vi "Main_20A.vi"() -> ()   [LabVIEW 2024]
uses:
  Utility/Universal Utility/TypeDefs_Utility/Cluster_Row-Column.ctl
  9e3f57c0-2ef8-4495-8287-c6a42a5fb955.vi
  Utility/Universal Utility/TypeDefs_Utility/ENUM_4 Directions U-D-L-R.ctl
  Utility/Universal Utility/TypeDefs_Utility/ENUM_8 Directions U-D-L-R.ctl
panel:
  in  "Select Data":enum32{"Example", "Puzzle"}(tab)
  in  "Example":string="###############\n#...#...#.....#\n#.#.#.#.#.###.#\n#S#...#.#.#...#\n#######.#.#.###\n#######.#.#...#\n#######.#.###.#\n###..E#...#...#\n###.#######.###\n#...###...#...#\n#.#####.#.###.#\n#.#...#.#.#...#\n#.#.#.#.#.#.###\n#...#...#...###\n###############"
  in  "Puzzle":string="#############################################################################################################################################\n#...............#...#...#.......#...#.........###...#...#.....#...#...........#...###.....###.....#.....#...###.........#...#...#...###.....#\n#.#############.#.#.#.#.#.#####.#.#.#.#######.###.#.#.#.#.###.#.#.#.#########.#.#.###.###.###.###.#.###.#.#.###.#######.#.#.#.#.#.#.###.###.#\n#.....#.......#.#.#...#.#.....#...#.#...#.....#...#.#.#...#...#.#.#.......#...#.#...#...#.#...#...#.#...#.#.#...#.......#.#.#.#.#.#...#...#.#\n#####.#.#####.#.#.#####.#####.#####.###.#.#####.###.#.#####.###.#.#######.#.###.###.###.#.#.###.###.#.###.#.#.###.#######.#.#.#.#.###.###.#.#\n#...#...#.....#...#...#.#...#.....#...#.#.....#...#...#.....#...#...###...#...#...#...#.#.#...#...#.#.#...#.#...#.....###.#.#.#...#...#...#.#\n#.#.#####.#########.#.#.#.#.#####.###.#.#####.###.#####.#####.#####.###.#####.###.###.#.#.###.###.#.#.#.###.###.#####.###.#.#.#####.###.###.#\n#.#.#...#.....#...#.#.#...#.#...#.#...#.....#...#...#...#...#.....#...#.....#...#.#...#.#.###...#.#.#...#...#...#.....#...#.#.#.....###...#.#\n#.#.#.#.#####.#.#.#.#.#####.#.#.#.#.#######.###.###.#.###.#.#####.###.#####.###.#.#.###.#.#####.#.#.#####.###.###.#####.###.#.#.#########.#.#\n#.#...#.#...#...#...#.....#.#.#.#.#.#...#...#...#...#...#.#.#.....#...###...#...#.#...#.#.#...#.#...#...#.#...#...#...#...#.#.#...#...#...#.#\n#.#####.#.#.#############.#.#.#.#.#.#.#.#.###.###.#####.#.#.#.#####.#####.###.###.###.#.#.#.#.#.#####.#.#.#.###.###.#.###.#.#.###.#.#.#.###.#\n#...#...#.#.#...#.....#...#...#...#.#.#.#...#...#.#...#...#.#...#...#...#.#...#...#...#.#.#.#.#.....#.#...#...#.###.#...#.#.#.#...#.#...#...#\n###.#.###.#.#.#.#.###.#.###########.#.#.###.###.#.#.#.#####.###.#.###.#.#.#.###.###.###.#.#.#.#####.#.#######.#.###.###.#.#.#.#.###.#####.###\n#...#.#...#.#.#.#...#.#...........#.#.#.###.#...#.#.#.......#...#...#.#.#.#.#...#...###.#.#.#.#...#.#...#.....#...#...#.#.#...#...#.....#...#\n#.###.#.###.#.#.###.#.###########.#.#.#.###.#.###.#.#########.#####.#.#.#.#.#.###.#####.#.#.#.#.#.#.###.#.#######.###.#.#.#######.#####.###.#\n#...#.#...#.#.#.#...#.#...........#...#...#.#...#.#.....#...#...#...#.#...#.#...#.###...#.#.#.#.#...#...#.....#...#...#...#.......#...#.#...#\n###.#.###.#.#.#.#.###.#.#################.#.###.#.#####.#.#.###.#.###.#####.###.#.###.###.#.#.#.#####.#######.#.###.#######.#######.#.#.#.###\n#...#...#.#.#.#.#...#.#...............#...#...#...#.....#.#.#...#...#.....#.....#...#...#.#.#.#...#...#...#...#...#...#.....#...#...#.#.#...#\n#.#####.#.#.#.#.###.#.###############.#.#####.#####.#####.#.#.#####.#####.#########.###.#.#.#.###.#.###.#.#.#####.###.#.#####.#.#.###.#.###.#\n#.....#...#.#.#.....#.###.............#.......#.....#...#.#.#.....#...###...#.....#.#...#.#.#...#.#.###.#.#.#.....###.#.....#.#.#...#.#.#...#\n#####.#####.#.#######.###.#####################.#####.#.#.#.#####.###.#####.#.###.#.#.###.#.###.#.#.###.#.#.#.#######.#####.#.#.###.#.#.#.###\n#...#.....#.#...#...#...#.....................#...###.#.#.#.#...#.#...#...#...#...#...#...#...#...#.....#.#.#...###...#...#...#.....#...#...#\n#.#.#####.#.###.#.#.###.#####################.###.###.#.#.#.#.#.#.#.###.#.#####.#######.#####.###########.#.###.###.###.#.#################.#\n#.#.....#.#.###...#...#...#...###...#...#...#...#.....#.#.#.#.#...#.###.#.#...#...#...#...#...#...........#...#.....#...#.......#.....#...#.#\n#.#####.#.#.#########.###.#.#.###.#.#.#.#.#.###.#######.#.#.#.#####.###.#.#.#.###.#.#.###.#.###.#############.#######.#########.#.###.#.#.#.#\n#.#...#...#...#...###...#.#.#.#...#.#.#...#...#...#.....#.#.#.....#...#.#...#.#...#.#.....#...#.........#...#.#.......###...###.#...#...#...#\n#.#.#.#######.#.#.#####.#.#.#.#.###.#.#######.###.#.#####.#.#####.###.#.#####.#.###.#########.#########.#.#.#.#.#########.#.###.###.#########\n#...#.....#...#.#.#.....#...#...#...#.......#.#...#.#...#.#...###.#...#.#.....#...#.#.....#...#.........#.#...#.#.......#.#...#...#.........#\n#########.#.###.#.#.#############.#########.#.#.###.#.#.#.###.###.#.###.#.#######.#.#.###.#.###.#########.#####.#.#####.#.###.###.#########.#\n#.........#...#.#.#...#.........#...###.....#.#...#.#.#...#...#...#.###.#.....###.#.#.#...#...#.....#...#.....#.#.#.....#.#...###...#.....#.#\n#.###########.#.#.###.#.#######.###.###.#####.###.#.#.#####.###.###.###.#####.###.#.#.#.#####.#####.#.#.#####.#.#.#.#####.#.#######.#.###.#.#\n#...........#...#.....#.#.....#...#.#...#...#.#...#.#.....#.#...#...#...#.....#...#.#.#...#...#...#.#.#...#...#.#.#.......#...###...#...#.#.#\n###########.###########.#.###.###.#.#.###.#.#.#.###.#####.#.#.###.###.###.#####.###.#.###.#.###.#.#.#.###.#.###.#.###########.###.#####.#.#.#\n#...#.......#...#...#...#...#.....#.#.#...#...#.#...#...#.#.#...#.###...#.#...#...#.#.#...#...#.#...#.#...#.#...#.#.........#...#.......#...#\n#.#.#.#######.#.#.#.#.#####.#######.#.#.#######.#.###.#.#.#.###.#.#####.#.#.#.###.#.#.#.#####.#.#####.#.###.#.###.#.#######.###.#############\n#.#.#.......#.#...#...#####...#...#...#.#...#...#...#.#.#.#.#...#.#.....#.#.#.#...#...#...#...#...#...#...#.#.#...#.......#...#.............#\n#.#.#######.#.###############.#.#.#####.#.#.#.#####.#.#.#.#.#.###.#.#####.#.#.#.#########.#.#####.#.#####.#.#.#.#########.###.#############.#\n#.#.........#.#.........#...#...#...###...#.#.....#.#.#...#.#.#...#.....#.#.#.#.###.......#...#...#...#...#.#...#...#...#...#...........#...#\n#.###########.#.#######.#.#.#######.#######.#####.#.#.#####.#.#.#######.#.#.#.#.###.#########.#.#####.#.###.#####.#.#.#.###.###########.#.###\n#...#...#...#.#.......#.#.#...#...#.....#...#.....#.#...#...#.#...#...#.#...#.#...#...#...#...#...#...#.....#.....#...#.....#...###...#...###\n###.#.#.#.#.#.#######.#.#.###.#.#.#####.#.###.#####.###.#.###.###.#.#.#.#####.###.###.#.#.#.#####.#.#########.###############.#.###.#.#######\n###...#...#...#.......#.#...#.#.#.#.....#...#...###...#.#...#...#.#.#.#...#...#...###...#.#...###.#.#...#...#...#...###.......#.....#...#...#\n###############.#######.###.#.#.#.#.#######.###.#####.#.###.###.#.#.#.###.#.###.#########.###.###.#.#.#.#.#.###.#.#.###.###############.#.#.#\n#...#...###...#.#.....#.....#...#...#...###...#...#...#.#...#...#.#.#.#...#...#.......###.....#...#.#.#...#.....#.#.....#.........#...#...#.#\n#.#.#.#.###.#.#.#.###.###############.#.#####.###.#.###.#.###.###.#.#.#.#####.#######.#########.###.#.###########.#######.#######.#.#.#####.#\n#.#.#.#.#...#.#.#.###.......#...#...#.#.....#.#...#.#...#...#...#.#.#.#.....#...#...#.#.....###.....#.............#...#...#...###...#.......#\n#.#.#.#.#.###.#.#.#########.#.#.#.#.#.#####.#.#.###.#.#####.###.#.#.#.#####.###.#.#.#.#.###.#######################.#.#.###.#.###############\n#.#.#.#.#.#...#...#...#...#...#...#...#.....#.#.#...#.#.....#...#.#.#...#...#...#.#.#...#...#...........#...#.......#...#...#...#...###...###\n#.#.#.#.#.#.#######.#.#.#.#############.#####.#.#.###.#.#####.###.#.###.#.###.###.#.#####.###.#########.#.#.#.###########.#####.#.#.###.#.###\n#.#...#...#...#.....#...#.............#.#...#...#...#.#.#...#...#.#.#...#...#...#.#...#...###.....#...#.#.#.#.............#.....#.#.....#...#\n#.###########.#.#####################.#.#.#.#######.#.#.#.#.###.#.#.#.#####.###.#.###.#.#########.#.#.#.#.#.###############.#####.#########.#\n#.......#...#...#...#...............#.#...#.....###.#.#...#.#...#...#...#...#...#.#...#...#...#...#.#.#...#...............#.......#.........#\n#######.#.#.#####.#.#.#############.#.#########.###.#.#####.#.#########.#.###.###.#.#####.#.#.#.###.#.###################.#########.#########\n#.......#.#.#...#.#.#.#.....###.....#.........#.#...#.#.....#.....#.....#...#...#.#...#...#.#...#...#.........#.........#.#...#...#.........#\n#.#######.#.#.#.#.#.#.#.###.###.#############.#.#.###.#.#########.#.#######.###.#.###.#.###.#####.###########.#.#######.#.#.#.#.#.#########.#\n#.#...#...#.#.#...#...#...#.....#...........#...#.#...#.#...#.....#...#...#...#...#...#...#.......#.........#...#.......#...#.#.#...#...#...#\n#.#.#.#.###.#.###########.#######.#########.#####.#.###.#.#.#.#######.#.#.###.#####.#####.#########.#######.#####.###########.#.###.#.#.#.###\n#.#.#.#...#...###...#...#.........#...#...#...###...#...#.#.#.......#...#.....#...#.......#...#...#.......#.......#...#...###...###.#.#.#...#\n#.#.#.###.#######.#.#.#.###########.#.#.#.###.#######.###.#.#######.###########.#.#########.#.#.#.#######.#########.#.#.#.#########.#.#.###.#\n#.#.#.....#.......#.#.#.###.........#...#.....#...###.....#.#.......###.......#.#.#...#.....#...#.#...###.........#.#...#.....#...#...#.....#\n#.#.#######.#######.#.#.###.###################.#.#########.#.#########.#####.#.#.#.#.#.#########.#.#.###########.#.#########.#.#.###########\n#...#.....#.......#.#.#...#.........#...#.......#.........#.#...#.....#.....#...#...#...#...#...#...#...#.......#...#...#...#...#.......#...#\n#####.###.#######.#.#.###.#########.#.#.#.###############.#.###.#.###.#####.#############.#.#.#.#######.#.#####.#####.#.#.#.###########.#.#.#\n#...#...#.###...#.#.#...#.#...#...#...#...#.....#.....#...#...#...#...###...#.....#...#...#...#.....#...#.#...#.......#...#.............#.#.#\n#.#.###.#.###.#.#.#.###.#.#.#.#.#.#########.###.#.###.#.#####.#####.#####.###.###.#.#.#.###########.#.###.#.#.###########################.#.#\n#.#...#.#.....#...#.....#...#.#.#.#.........###...###.#.....#.#...#.....#...#.###...#.#.###.........#.....#.#.###...###...................#.#\n#.###.#.#####################.#.#.#.#################.#####.#.#.#.#####.###.#.#######.#.###.###############.#.###.#.###.###################.#\n#...#.#.......#.....#...#...#...#...###.............#...#...#...#.....#.#...#.#.......#...#...#.......#.....#.....#...#.#.........#.........#\n###.#.#######.#.###.#.#.#.#.###########.###########.###.#.###########.#.#.###.#.#########.###.#.#####.#.#############.#.#.#######.#.#########\n#...#...#...#.#.###.#.#...#.............#.......#...###.#.....#...#...#.#.....#...........###...###...#.#...........#...#.......#.#.#...#...#\n#.#####.#.#.#.#.###.#.###################.#####.#.#####.#####.#.#.#.###.###########################.###.#.#########.###########.#.#.#.#.#.#.#\n#.....#...#...#.#...#...#...............#.#...#...#...#.......#.#.#.....#E............#...#...#...#.....#.#.......#.#...........#...#.#.#.#.#\n#####.#########.#.#####.#.#############.#.#.#.#####.#.#########.#.###################.#.#.#.#.#.#.#######.#.#####.#.#.###############.#.#.#.#\n#.....#.....#...#.....#.#.............#.#...#.......#.......#...#...#...#############...#...#...#.......#...#...#.#.#.#.......#...#...#...#.#\n#.#####.###.#.#######.#.#############.#.###################.#.#####.#.#.###############################.#####.#.#.#.#.#.#####.#.#.#.#######.#\n#.#.....###...#...###.#.#.............#...#.............#...#...#...#.#.....###########################.......#.#.#.#...#.....#.#...#...#...#\n#.#.###########.#.###.#.#.###############.#.###########.#.#####.#.###.#####.###################################.#.#.#####.#####.#####.#.#.###\n#...#...........#...#...#...........#...#.#...........#.#...###.#...#...#...###################################...#.#...#...###.#.....#...###\n#####.#############.###############.#.#.#.###########.#.###.###.###.###.#.#########################################.#.#.###.###.#.###########\n#.....#...........#.###...#...#...#...#.#.#...........#.....#...#...#...#...#######################################...#.....#...#...........#\n#.#####.#########.#.###.#.#.#.#.#.#####.#.#.#################.###.###.#####.#################################################.#############.#\n#...#...#.........#.....#...#...#.....#.#.#.###...#.....#...#...#.###.....#.....#####################.....#########.....###...#...#.......#.#\n###.#.###.###########################.#.#.#.###.#.#.###.#.#.###.#.#######.#####.#####################.###.#########.###.###.###.#.#.#####.#.#\n###...###...#...#.....#...#.........#...#...#...#...#...#.#.#...#.....#...#.....#####....S#.....#...#...#.....#####...#...#...#.#...#...#...#\n###########.#.#.#.###.#.#.#.#######.#########.#######.###.#.#.#######.#.###.#########.#####.###.#.#.###.#####.#######.###.###.#.#####.#.#####\n#.......###.#.#.#.###...#...#...###.........#.#.......#...#.#.....#...#...#.#...#####.....#.###...#.....#.....###...#...#...#.#.....#.#.....#\n#.#####.###.#.#.#.###########.#.###########.#.#.#######.###.#####.#.#####.#.#.#.#########.#.#############.#######.#.###.###.#.#####.#.#####.#\n#.#...#.....#.#.#.#...........#.......#...#...#...#...#...#.#...#.#.#...#.#...#.#####.....#.#...#.....#...#.....#.#.#...#...#.#.....#.#.....#\n#.#.#.#######.#.#.#.#################.#.#.#######.#.#.###.#.#.#.#.#.#.#.#.#####.#####.#####.#.#.#.###.#.###.###.#.#.#.###.###.#.#####.#.#####\n#.#.#.....#...#...#.........#.......#...#.........#.#.....#.#.#...#.#.#.#.#.....#####...#...#.#.#...#.#.....#...#.#.#...#.....#.......#.#...#\n#.#.#####.#.###############.#.#####.###############.#######.#.#####.#.#.#.#.###########.#.###.#.###.#.#######.###.#.###.###############.#.#.#\n#...#.....#.#.....#...#.....#.#.....#.........###...#.....#.#.#...#.#.#.#.#.....###...#...#...#.....#.........#...#.....#...#...#.....#...#.#\n#####.#####.#.###.#.#.#.#####.#.#####.#######.###.###.###.#.#.#.#.#.#.#.#.#####.###.#.#####.###################.#########.#.#.#.#.###.#####.#\n#.....#...#.#...#...#...#.....#.......#.......#...#...###...#...#.#.#.#.#.#...#.#...#.....#.#...#.....#...#.....#...#.....#...#...###.......#\n#.#####.#.#.###.#########.#############.#######.###.#############.#.#.#.#.#.#.#.#.#######.#.#.#.#.###.#.#.#.#####.#.#.#######################\n#...#...#...###...........#...........#.....###...#.....#...###...#.#.#.#.#.#...#.......#.#...#...###...#...#.....#...#...#.........#.......#\n###.#.#####################.#########.#####.#####.#####.#.#.###.###.#.#.#.#.###########.#.###################.#########.#.#.#######.#.#####.#\n#...#.#.....#...#...........#.......#.....#.#.....#.....#.#.#...#...#.#.#.#...#...#.....#.###.........#.......#.........#...#.......#.#.....#\n#.###.#.###.#.#.#.###########.#####.#####.#.#.#####.#####.#.#.###.###.#.#.###.#.#.#.#####.###.#######.#.#######.#############.#######.#.#####\n#...#.#...#...#...#...........#.....#...#...#.....#.#...#.#.#.#...#...#.#.#...#.#.#.....#...#.......#.#.........#.....#.......###...#.#.#...#\n###.#.###.#########.###########.#####.#.#########.#.#.#.#.#.#.#.###.###.#.#.###.#.#####.###.#######.#.###########.###.#.#########.#.#.#.#.#.#\n#...#.#...#...#...#.#.........#.....#.#...#...#...#...#.#.#.#.#.###...#.#.#.#...#.#...#...#...#...#.#.#...........###...#.........#...#...#.#\n#.###.#.###.#.#.#.#.#.#######.#####.#.###.#.#.#.#######.#.#.#.#.#####.#.#.#.#.###.#.#.###.###.#.#.#.#.#.#################.#################.#\n#.....#.....#...#...#.......#.#...#.#.#...#.#.#.......#.#.#.#.#.#...#.#.#.#.#...#.#.#.###.#...#.#.#.#.#.........#...#.....#.................#\n###########################.#.#.#.#.#.#.###.#.#######.#.#.#.#.#.#.#.#.#.#.#.###.#.#.#.###.#.###.#.#.#.#########.#.#.#.#####.#################\n#...................#.......#...#...#.#...#.#.#...#...#...#...#.#.#...#.#.#.#...#.#.#.#...#...#.#.#.#.....#...#...#...#...#.............#...#\n#.#################.#.###############.###.#.#.#.#.#.###########.#.#####.#.#.#.###.#.#.#.#####.#.#.#.#####.#.#.#########.#.#############.#.#.#\n#.................#.#.............#...#...#.#.#.#.#.......#.....#.....#.#.#.#.#...#.#...###...#.#.#.....#.#.#.#.....#...#.#.......#.....#.#.#\n#################.#.#############.#.###.###.#.#.#.#######.#.#########.#.#.#.#.#.###.#######.###.#.#####.#.#.#.#.###.#.###.#.#####.#.#####.#.#\n#.........#...#...#...............#...#.#...#.#.#...#...#.#...#...#...#.#.#.#.#...#.......#.....#.#.....#.#.#.#...#.#...#...#...#...###...#.#\n#.#######.#.#.#.#####################.#.#.###.#.###.#.#.#.###.#.#.#.###.#.#.#.###.#######.#######.#.#####.#.#.###.#.###.#####.#.#######.###.#\n#.......#...#.#...........#.....#...#.#.#.#...#...#...#.#.#...#.#.#.#...#.#.#...#.#...#...#.......#.....#.#.#.#...#...#.......#.......#...#.#\n#######.#####.###########.#.###.#.#.#.#.#.#.#####.#####.#.#.###.#.#.#.###.#.###.#.#.#.#.###.###########.#.#.#.#.#####.###############.###.#.#\n#.......#...#.............#.###.#.#.#.#.#.#.#...#...#...#.#.#...#.#.#.....#...#.#...#.#...#.#.....#...#.#.#.#.#.....#.#.....#.........#...#.#\n#.#######.#.###############.###.#.#.#.#.#.#.#.#.###.#.###.#.#.###.#.#########.#.#####.###.#.#.###.#.#.#.#.#.#.#####.#.#.###.#.#########.###.#\n#.....#...#.................#...#.#.#.#.#.#.#.#.#...#...#.#.#.#...#.......###.#.#.....#...#.#...#.#.#...#.#.#.#.....#.#.#...#.........#...#.#\n#####.#.#####################.###.#.#.#.#.#.#.#.#.#####.#.#.#.#.#########.###.#.#.#####.###.###.#.#.#####.#.#.#.#####.#.#.###########.###.#.#\n#...#...#.....................#...#.#.#.#.#.#.#.#.....#...#...#.....#...#...#.#.#.....#...#...#.#.#.###...#.#.#...#...#.#.#...........#...#.#\n#.#.#####.#####################.###.#.#.#.#.#.#.#####.#############.#.#.###.#.#.#####.###.###.#.#.#.###.###.#.###.#.###.#.#.###########.###.#\n#.#...###.....#.....#...#...#...#...#.#.#.#.#.#.....#.#...#...#...#.#.#.....#...#.....#...#...#.#.#...#...#.#.....#.#...#.#.........#...#...#\n#.###.#######.#.###.#.#.#.#.#.###.###.#.#.#.#.#####.#.#.#.#.#.#.#.#.#.###########.#####.###.###.#.###.###.#.#######.#.###.#########.#.###.###\n#...#.........#...#...#.#.#.#...#.#...#.#.#.#...###.#...#.#.#...#...#...#...#...#...#...#...#...#.#...#...#.......#...#...#...#...#...#...###\n###.#############.#####.#.#.###.#.#.###.#.#.###.###.#####.#.###########.#.#.#.#.###.#.###.###.###.#.###.#########.#####.###.#.#.#.#####.#####\n#...#.....#.....#.#.....#.#...#.#...###.#.#.#...#...#...#.#.#.....#...#...#...#.#...#...#...#.#...#...#.#...#...#.#.....#...#.#.#.#...#.....#\n#.###.###.#.###.#.#.#####.###.#.#######.#.#.#.###.###.#.#.#.#.###.#.#.#########.#.#####.###.#.#.#####.#.#.#.#.#.#.#.#####.###.#.#.#.#.#####.#\n#.#...#...#.###...#.....#.###.#...#.....#.#...###...#.#...#.#.#...#.#...#.....#.#.#.....###.#.#.#...#.#.#.#.#.#.#.#.#...#...#...#.#.#.......#\n#.#.###.###.###########.#.###.###.#.#####.#########.#.#####.#.#.###.###.#.###.#.#.#.#######.#.#.#.#.#.#.#.#.#.#.#.#.#.#.###.#####.#.#########\n#.#...#...#.#...........#.#...#...#...#...###.......#.#...#...#...#...#.#.#...#.#.#...#...#...#.#.#.#.#.#.#...#...#...#.#...###...#...###...#\n#.###.###.#.#.###########.#.###.#####.#.#####.#######.#.#.#######.###.#.#.#.###.#.###.#.#.#####.#.#.#.#.#.#############.#.#####.#####.###.#.#\n#.#...###...#...........#.#...#.###...#.....#...#...#...#...#...#.#...#.#.#.#...#...#...#.#.....#.#.#.#.#.........#.....#...#...#...#.....#.#\n#.#.###################.#.###.#.###.#######.###.#.#.#######.#.#.#.#.###.#.#.#.#####.#####.#.#####.#.#.#.#########.#.#######.#.###.#.#######.#\n#.#.#.....#.............#.#...#...#.#...#...###...#...#...#...#.#.#.#...#.#.#.#...#.#.....#.#...#.#.#.#.#.....#...#.....#...#.#...#.#.....#.#\n#.#.#.###.#.#############.#.#####.#.#.#.#.###########.#.#.#####.#.#.#.###.#.#.#.#.#.#.#####.#.#.#.#.#.#.#.###.#.#######.#.###.#.###.#.###.#.#\n#.#.#...#...#...........#.#...#...#.#.#.#.###.........#.#.#...#.#...#...#.#.#.#.#...#.....#.#.#...#.#.#.#...#.#.#...#...#...#.#.###.#...#.#.#\n#.#.###.#####.#########.#.###.#.###.#.#.#.###.#########.#.#.#.#.#######.#.#.#.#.#########.#.#.#####.#.#.###.#.#.#.#.#.#####.#.#.###.###.#.#.#\n#...###.......#...#.....#...#.#...#.#.#.#...#.......#...#.#.#.#.....###...#.#.#.......#...#.#...###...#.#...#...#.#...#.....#...#...#...#.#.#\n###############.#.#.#######.#.###.#.#.#.###.#######.#.###.#.#.#####.#######.#.#######.#.###.###.#######.#.#######.#####.#########.###.###.#.#\n#...............#...#.....#.#...#.#.#.#.#...#.......#.#...#.#.#...#.......#.#.#.......#...#.#...#.......#.......#...#...#.........#...#...#.#\n#.###################.###.#.###.#.#.#.#.#.###.#######.#.###.#.#.#.#######.#.#.#.#########.#.#.###.#############.###.#.###.#########.###.###.#\n#.....................###...###...#...#...###.........#.....#...#.........#...#...........#...###...............###...###...........###.....#\n#############################################################################################################################################"
  out "Answer":u32
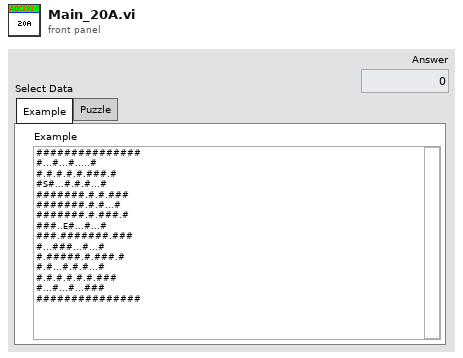
[diagram p1: front panel]
types:
  T1 = typedef "ENUM_8 Directions U-D-L-R.ctl" = enum16{"Up;-1,0", "Up-Right;-1,1", "Right;0,1", "Down-Right;1,1", "Down;1,0", "Down-Left;1,-1", "Left;0,-1", "Up-Left;-1,-1"}
  T2 = typedef "ENUM_4 Directions U-D-L-R.ctl" = enum16{"Up;-1,0", "Right;0,1", "Down;1,0", "Left;0,-1"}
  T3 = typedef "Cluster_Row-Column.ctl" = cluster{"R":i32, "C":i32}
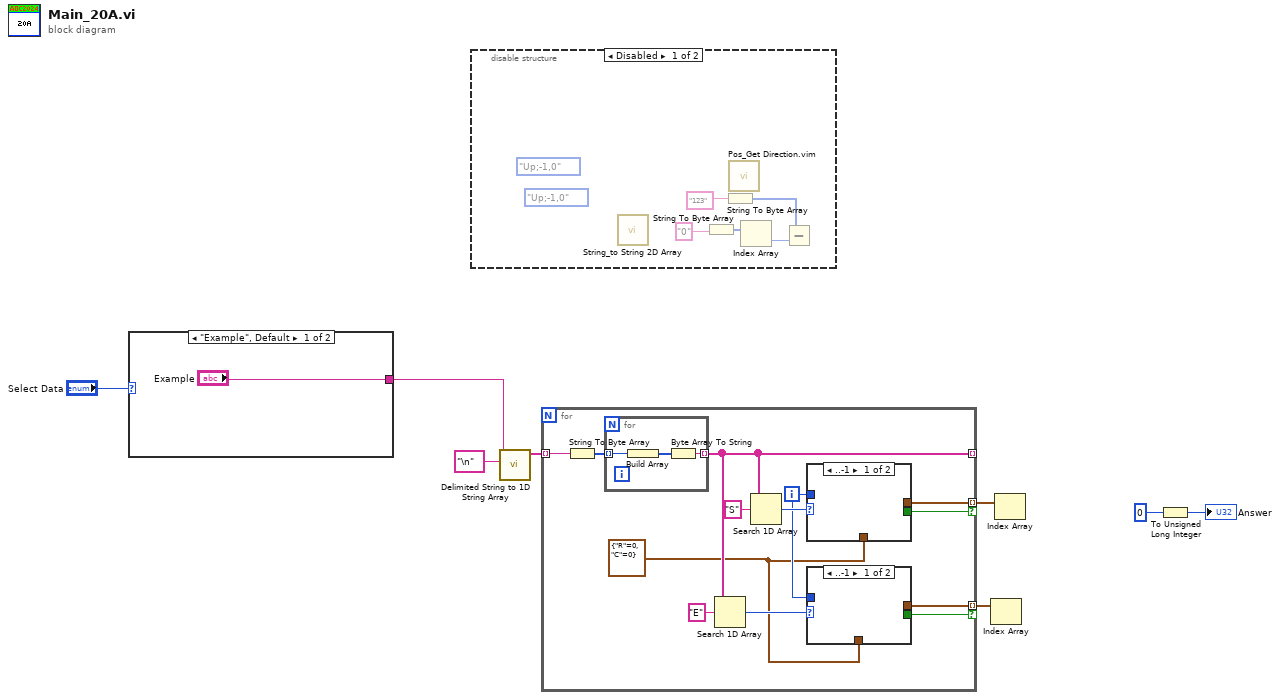
[diagram p0: block diagram]
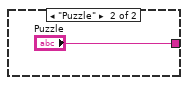
[diagram p2: hidden frame]
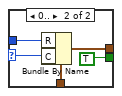
[diagram p4: hidden frame]
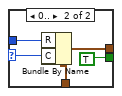
[diagram p5: hidden frame]
diagram:
  n1 = case shown="\"Example\", Default" "Select Data" {
    tunnel: ["Example" "Puzzle"] -> w3
    frame "Example", Default {
    }
    frame "Puzzle" {
    }
  }
  n2 = disable-structure shown="Disabled" {
    frame Disabled {
      (unwired) ENUM_8_Directions_U-D-L-R."Up;-1,0" ("Direction 8")
      (unwired) ENUM_4_Directions_U-D-L-R."Up;-1,0" ("Direction")
      n3 = call "String_to String 2D Array.vi"() -> ()  [unwired: 11 in, 1 out]
      n4 = String To Byte Array(string="0") -> (unsigned byte array=w13:u8[])
      n5 = String To Byte Array(string="123") -> (unsigned byte array=w11:u8[])
      n6 = call "Pos_Get Direction.vim"() -> ()  [unwired: 11 in, 1 out]
      n7 = Index Array(array=w13) -> (element=w12:u8)  [unwired: 1 in]
      n8 = Subtract(x=w11, y=w12) -> ()  [unwired: 1 out]
    }
    frame Enabled {
    }
  }
  n9 = call <vilib>:"Delimited String to 1D String Array.vi"("delimiter"="\n" ("delimiter (Tab)"), "delimited string"=w3) -> ("string array"=w7:string[])  [unwired: 9 in]
  n10 = for {
    tunnel: w7 -> [w27] mode=indexing
    tunnel: [w26] -> _ mode=indexing
    tunnel: [w22] -> w2 mode=indexing if=w21
    tunnel: [w17] -> w1 mode=indexing if=w16
    i -> [w20]
    w18 = T3 {"R"=0, "C"=0} ("Position")
    n11 = String To Byte Array(string=w27) -> (unsigned byte array=w28:u8[])
    n12 = for {
      tunnel: w28 -> [w41] mode=indexing
      tunnel: [w39] -> w26 mode=indexing
      n13 = Build Array(w41) -> (w40:u8[])
      n14 = Byte Array To String(unsigned byte array=w40) -> (string=w39:string)
    }
    n15 = Search 1D Array(1D array=w26, element="E") -> (index of element=w19:i32)  [unwired: 1 in]
    n16 = Search 1D Array(1D array=w26, element="S") -> (index of element=w23:i32)  [unwired: 1 in]
    n17 = case shown="..-1" w23 {
      selector: w23 -> [_ w36]
      tunnel: w20 -> [_ w37]
      tunnel: w18 -> [_ w38]
      tunnel: [_ w35] -> w22
      tunnel: [_ TRUE] -> w21
      frame ..-1 {
      }
      frame 0.. {
        n18 = Bundle By Name(cluster=w38, "R"=w37, "C"=w36) -> (w35:T3)
      }
    }
    n19 = case shown="..-1" w19 {
      selector: w19 -> [_ w31]
      tunnel: w20 -> [_ w32]
      tunnel: w18 -> [_ w33]
      tunnel: [_ w30] -> w17
      tunnel: [_ TRUE] -> w16
      frame ..-1 {
      }
      frame 0.. {
        n20 = Bundle By Name(cluster=w33, "R"=w32, "C"=w31) -> (w30:T3)
      }
    }
  }
  n21 = Index Array(array=w1) -> ()  [unwired: 1 in, 1 out]
  n22 = Index Array(array=w2) -> ()  [unwired: 1 in, 1 out]
  n23 = To Unsigned Long Integer(number=u32 0) -> (unsigned 32bit integer=→"Answer":u32)
